vi "parseDescription.vi"(6 "Deleted Rows":string[][](array[string]), 10 "Ch names Out":string[](array[string])) -> (1 "values":u32[](array[numeric]), 2 "titles":string[](array[string])=["Rows:logged:n", "message:Length:chars", "errors:Unique:n", "errors:Total:n"])   [LabVIEW 2020]
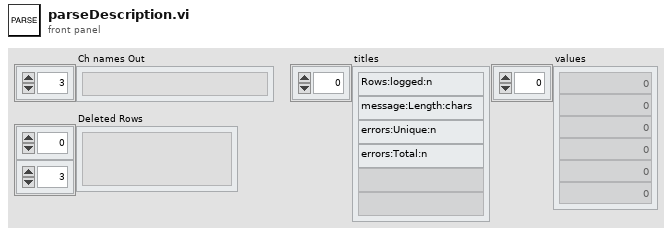
[diagram p1: front panel]
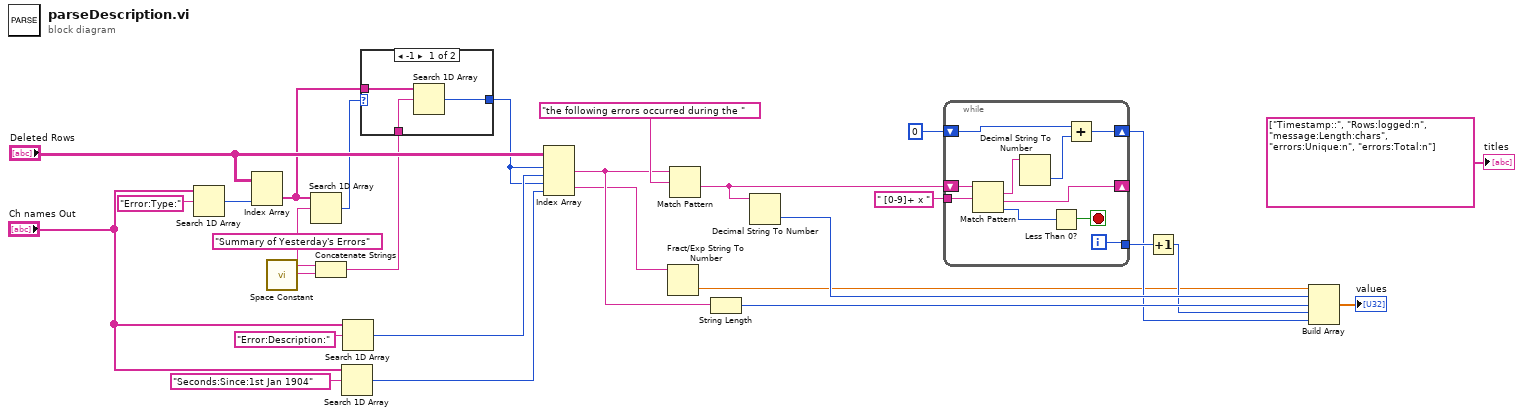
[diagram p0: block diagram]
diagram:
  w4 = "Summary of Yesterday's Errors" ("String")
  n1 = Search 1D Array(1D array="Ch names Out", element="Error:Type:" ("String")) -> (index of element=w25:i32)  [unwired: 1 in]
  n2 = Index Array(array="Deleted Rows", index (col)=w25) -> (element=w2:string[])  [unwired: 1 in]
  n3 = call <vilib>:"Space Constant.vi"() -> ("String"=w3:string)
  n4 = Search 1D Array(1D array=w2, element=w4) -> (index of element=w6:i32)  [unwired: 1 in]
  n5 = Concatenate Strings(w4, w3) -> (w1:string)
  n6 = Search 1D Array(1D array="Ch names Out", element="Seconds:Since:1st Jan 1904" ("String")) -> (index of element=w9:i32)  [unwired: 1 in]
  n7 = Search 1D Array(1D array="Ch names Out", element="Error:Description:" ("String")) -> (index of element=w28:i32)  [unwired: 1 in]
  n8 = case shown="-1" w6 {
    selector: w6 -> [_ w32]
    tunnel: [w29 w32] -> w5
    tunnel: w2 -> [w31 _]
    tunnel: w1 -> [w30 _]
    frame -1 {
      n9 = Search 1D Array(1D array=w31, element=w30) -> (index of element=w29:i32)  [unwired: 1 in]
    }
    frame 1, Default {
    }
  }
  n10 = Index Array(array="Deleted Rows", index (row) #1=w5, index (col) #1=w28, index (row) #2=w5, index (col) #2=w9) -> (element #1=w22:string, element #2=w8:string)
  n11 = Fract/Exp String To Number(string=w8) -> (number=w7:dbl)  [unwired: 3 in, 1 out]
  n12 = Match Pattern(string=w22, regular expression="the following errors occurred during the " ("format string")) -> (after substring=w21:string)  [unwired: 1 in, 3 out]
  n13 = String Length(string=w22) -> (length=w15:i32)
  n14 = Decimal String To Number(string=w21) -> (number=w16:i32)  [unwired: 2 in, 1 out]
  n15 = while {
    shift-right: [w41] -> _
    shift-left: w21 -> [w42]
    shift-right: [w39] -> w13
    shift-left: 0 -> [w40]
    tunnel: " [0-9]+ x " ("regular expression") -> [w36]
    tunnel: [w33] -> w18
    i -> [w33]
    stop <- w35 stop-if-true
    n16 = Match Pattern(string=w42, regular expression=w36) -> (match substring=w34:string, after substring=w41:string, offset past match=w37:i32)  [unwired: 1 in, 1 out]
    n17 = Decimal String To Number(string=w34) -> (number=w38:i32)  [unwired: 2 in, 1 out]
    n18 = Less Than 0?(x=w37) -> (x < 0?=w35:bool)
    n19 = Add(x=w40, y=w38) -> (x+y=w39:i32)
  }
  n20 = Increment(x=w18) -> (x+1=w14:i32)
  n21 = Build Array(w7, w16, w15, w14, w13) -> (→"values":dbl[])
  "titles" <- string[] ["Timestamp::", "Rows:logged:n", "message:Length:chars", "errors:Unique:n", "errors:Total:n"]
